vi "Calib_Inst_ch_info.vi"(1 "Input string":string) -> (0 "instrument to calibrate":T1(array[cluster])=[{"Ch No"=1, "Off ch no"=1, "Device"="", "Port"=""}, {"Ch No"=2, "Off ch no"=1, "Device"="", "Port"=""}] {"Off ch no" min=0 max=1; "Ch No" min=0 max=7})   [LabVIEW 2022 SP3]
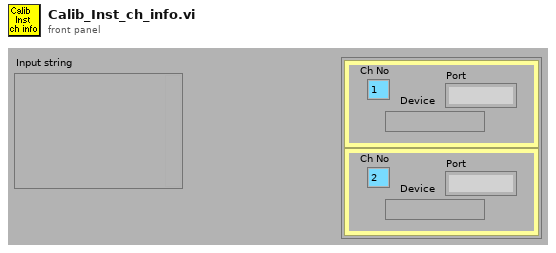
[diagram p1: front panel]
types:
  T1 = cluster{"Ch No":i16, "Off ch no":i8, "Device":string, "Port":string}[]
  T2 = cluster{"Ch No":i16, "Off ch no":i8, "Device":string, "Port":string}
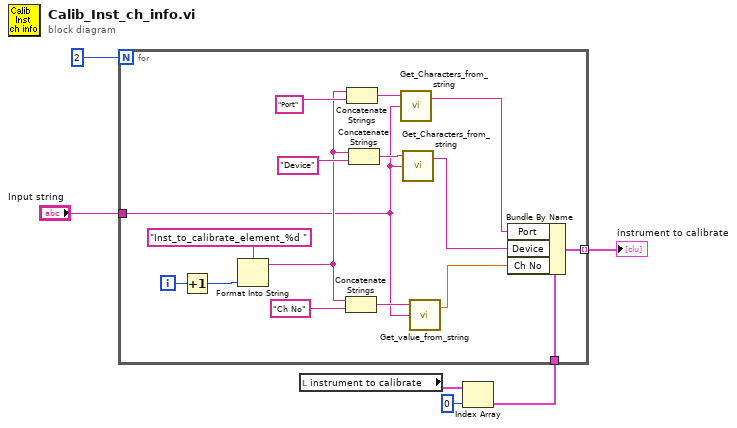
[diagram p0: block diagram]
diagram:
  n1 = local read "instrument to calibrate"() -> (w3:T1)
  n2 = Index Array(array=w3, index=0) -> (element=w1:T2)
  n3 = for {
    N: 2 -> [_]
    tunnel: w1 -> [w18]
    tunnel: "Input string" -> [w8]
    tunnel: [w15] -> w5 mode=indexing
    i -> [w22]
    n4 = Increment(x=w22) -> (x+1=w20:i32)
    n5 = Format Into String(format string="Inst_to_calibrate_element_%d ", w20) -> (resulting string=w9:string)  [unwired: 2 in, 1 out]
    n6 = Concatenate Strings(w9, "Ch No") -> (w17:string)
    n7 = Concatenate Strings(w9, "Port") -> (w11:string)
    n8 = Concatenate Strings(w9, "Device") -> (w13:string)
    n9 = call "Get_Characters_from_string.vi"("Input string"=w8, "Variable name"=w11) -> ("Value"=w7:string)  [unwired: 1 in, 1 out]
    n10 = call "Get_Characters_from_string.vi"("Input string"=w8, "Variable name"=w13) -> ("Value"=w12:string)  [unwired: 1 in, 1 out]
    n11 = call "Get_value_from_string.vi"("Input string"=w8, "Variable name"=w17) -> ("Value"=w16:dbl)  [unwired: 1 in, 1 out]
    n12 = Bundle By Name(cluster=w18, "Port"=w7, "Device"=w12, "Ch No"=w16) -> (w15:T2)
  }
  "instrument to calibrate" <- w5
